vi "Reshape volume imaging data.vi"(0 "tdms file ref":refnum<k34>, 1 "TDMS file path & name":path=path "C:/Users/Theo/Desktop/Datasets/140401_17_44_08-rig 3 debugging/Functional imaging TDMS data files/001.tdms", 5 "All header parameters":T1={"Imaging Protocol"=enum."AOL Z-Stack", "Number of POI"=0, "Number of Miniscans"=0, "Number of Trials"=0, "Number of Cycles "=0, "# Averaged Frames"=0, "Laser power (%)"=0, "Pockels"=0.0, "Acquisition Length (sec)"=0.0, "Fill time (us)"=0.0, "POI Dwell time (us)"=0.0, "Miniscan Dwell time per pixel (us)"=0.0, "PMT 1"=0.0, "PMT 2"=0.0, "Back Apperture"=0.0, "Zoom"=0.0, "Frame Size"=200, "Center Frequency"=0.0, "Field of View"=0.0, "DwellTime (us)"=0.0, "Wavelength (nm)"=0.0, "AOL Z"=0.0, "AOL Mode"=enum."Raster", "GridXY"=0.0, "GridZ"=0.0, "TriggerDelay (sec)"=0.0, "Number of Pixels in Miniscan"=0, "Experiment folder path"=path "", "X centre"=0.0, "Y centre"=0.0, "Angle (degrees)"=0.0, "Plane Mode"=0, "Software version"=0.0, "Objective"="Olympus  20X", "MotorZ Calibration"=0, "Pockels Calibration"=0, "Threshold"=[], "Video length (sec)"=0.0, "Frame rate (fps)"=0, "Rectangle ROI length (pixels)"=0, "Rectangle ROI height (pixels)"=0} {"Pockels" format="%#.6g"; "Software version" format="%#.6g"; "Plane Mode" items=["XY Plane"]; "Angle (degrees)" format="%#.6g"; "Frame Size" items=["100X100"=100, "128X128"=128, "200X200"=200, "256X256"=256, "512X512"=512, "1024x1024"=1024, "2048x2048"=2048]; "Back Apperture" format="%#.6g"; "PMT 2" format="%#.6g"; "PMT 1" format="%#.6g"; "Miniscan Dwell time per pixel (us)" format="%#.6g"; "Zoom" format="%#.6g"; "POI Dwell time (us)" format="%#.6g"; "Acquisition Length (sec)" format="%#.6g"; "Fill time (us)" format="%#.6g"}, 11 "error in (no error)":errorcluster, 12 "Channel to process":enum16{"Red", "Green", "Both"}(ring)) -> (4 "tdms file out":refnum<k34>, 6 "Single channel data":u16[](array[numeric]), 8 "Channel 4D data":u16[][][][](array[numeric]), 10 "Volumetric parameters":T7, 14 "Angles (deg)":dbl[](array[numeric]), 15 "error out":errorcluster)   [LabVIEW 2013]
uses:
  User Interface/Visualisation/Functional Imaging Viewer/SubVIs/Experiment header interface/Typedefs/Header parameters cluster-ALL.ctl
  Typedefs/Imaging Protocols enum.ctl
  Typedefs/Frame Size.ctl
  Typedefs/AOL modes.ctl
  Typedefs/Plane Mode.ctl
  Typedefs/Objective selector control enum.ctl
panel:
  out "Points in each volume or trial (fractional)":dbl
  out "Points Mismatch":bool
  out "Resulting number of points":i32
  out "Points in each volume or trial":i32
  out "Points in all volumes":i32
  out "Channel size(s)":i32[](array[numeric])
  # "<---This should be an integer. If it is not review the logic inside this VI is suitable"
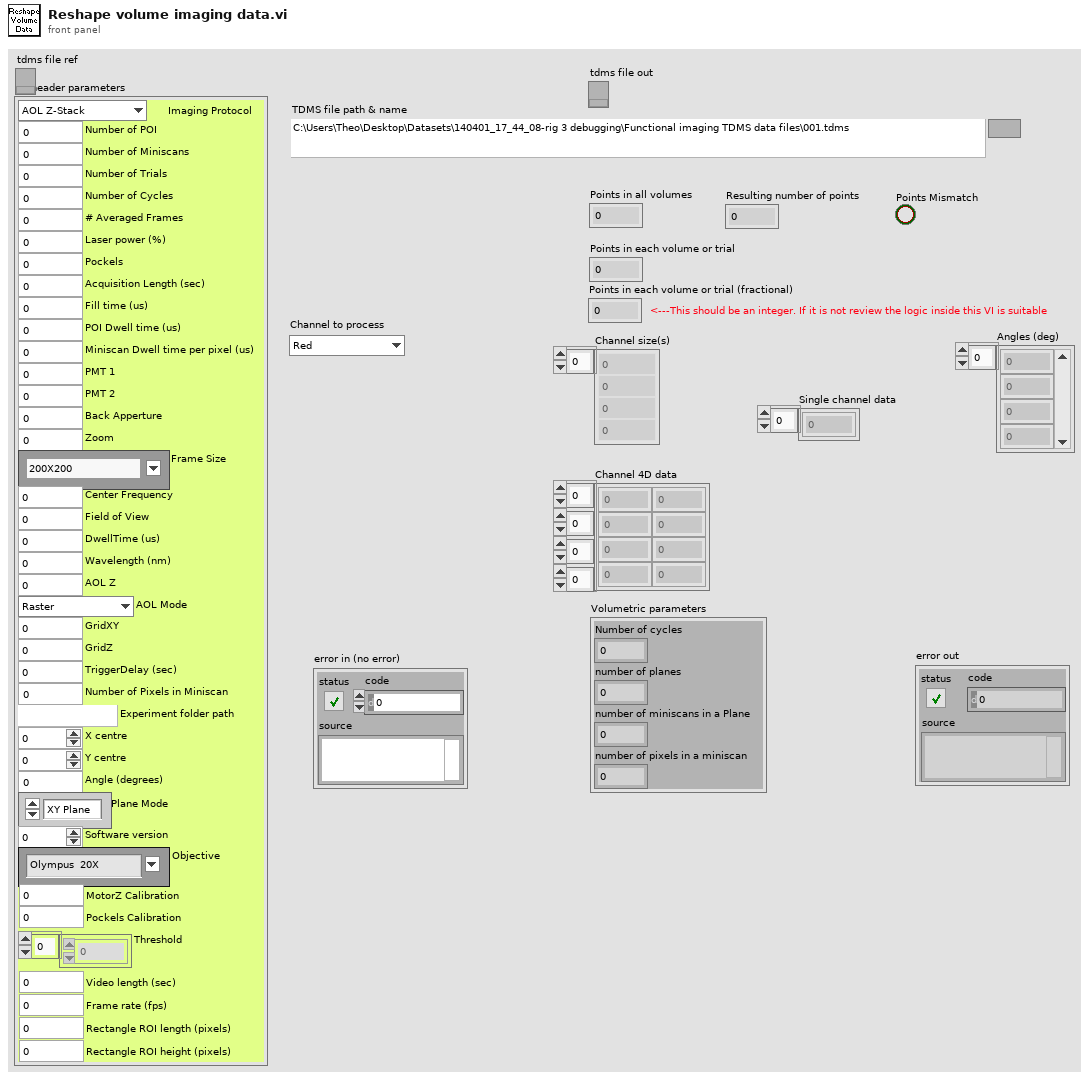
[diagram p1: front panel]
types:
  T1 = typedef "Header parameters cluster-ALL.ctl" = cluster{"Imaging Protocol":T2, "Number of POI":u16, "Number of Miniscans":u16, "Number of Trials":u16, "Number of Cycles ":u64, "# Averaged Frames":u16, "Laser power (%)":u8, "Pockels":dbl, "Acquisition Length (sec)":dbl, "Fill time (us)":dbl, "POI Dwell time (us)":dbl, "Miniscan Dwell time per pixel (us)":dbl, "PMT 1":dbl, "PMT 2":dbl, "Back Apperture":dbl, "Zoom":dbl, "Frame Size":T3, "Center Frequency":dbl, "Field of View":dbl, "DwellTime (us)":dbl, "Wavelength (nm)":dbl, "AOL Z":dbl, "AOL Mode":T4, "GridXY":dbl, "GridZ":dbl, "TriggerDelay (sec)":dbl, "Number of Pixels in Miniscan":u16, "Experiment folder path":path, "X centre":dbl, "Y centre":dbl, "Angle (degrees)":dbl, "Plane Mode":T5, "Software version":dbl, "Objective":T6, "MotorZ Calibration":u32, "Pockels Calibration":u32, "Threshold":u16[], "Video length (sec)":dbl, "Frame rate (fps)":u8, "Rectangle ROI length (pixels)":u16, "Rectangle ROI height (pixels)":u16}
  T2 = typedef "Imaging Protocols enum.ctl" = enum16{"AOL Z-Stack", "Motor Z Stack", "Functional Acquisition", "Single Plane Acquisition", "Volume Acquisition", "Live Imaging", "Live Plane Imaging", "Live Volume Imaging"}
  T3 = typedef "Frame Size.ctl" = u16
  T4 = typedef "AOL modes.ctl" = enum16{"Raster", "Structural", "Pointing", "Mini Scan", "Alignment"}
  T5 = typedef "Plane Mode.ctl" = u16
  T6 = typedef "Objective selector control enum.ctl" = string
  T7 = cluster{"Number of cycles":i32, "number of planes":i32, "number of miniscans in a Plane":i32, "number of pixels in a miniscan":i32}
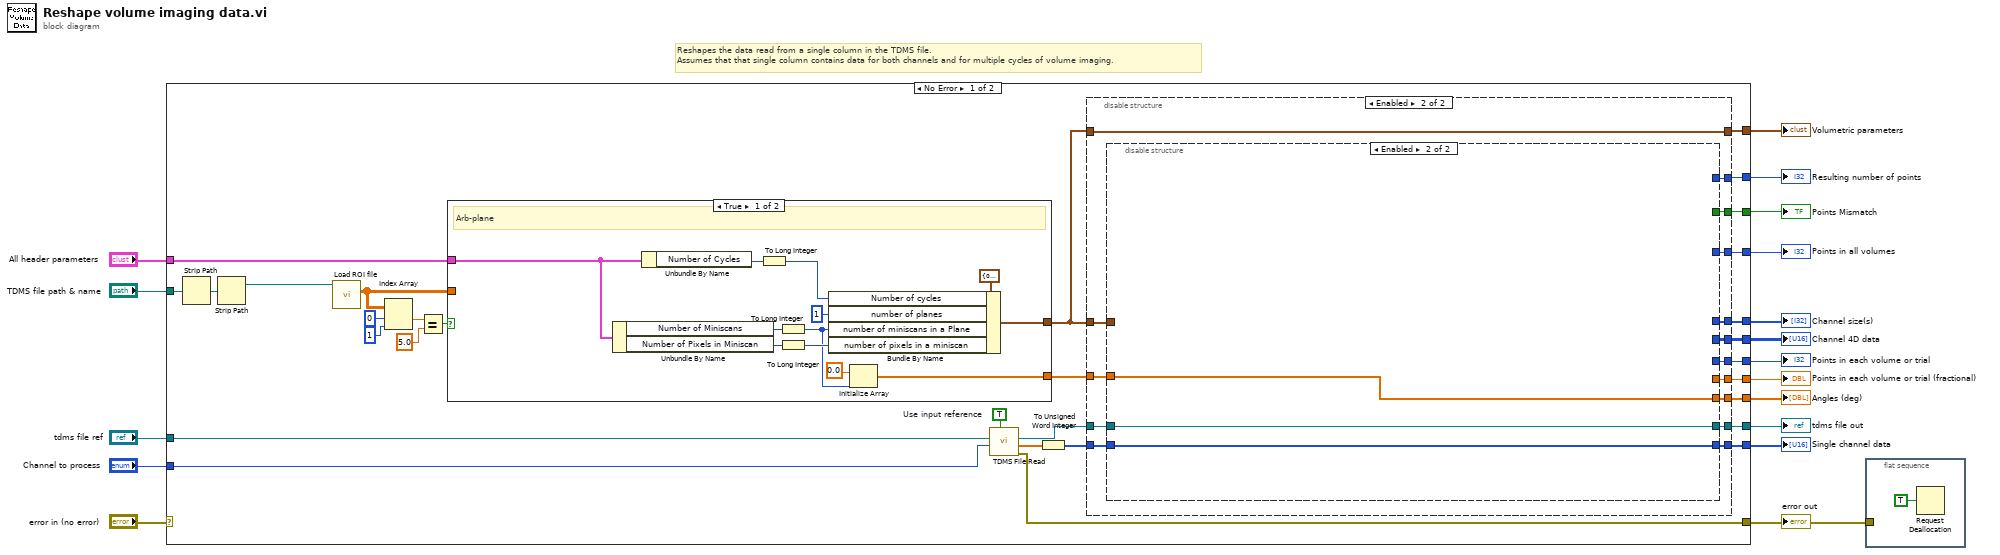
[diagram p0: block diagram]
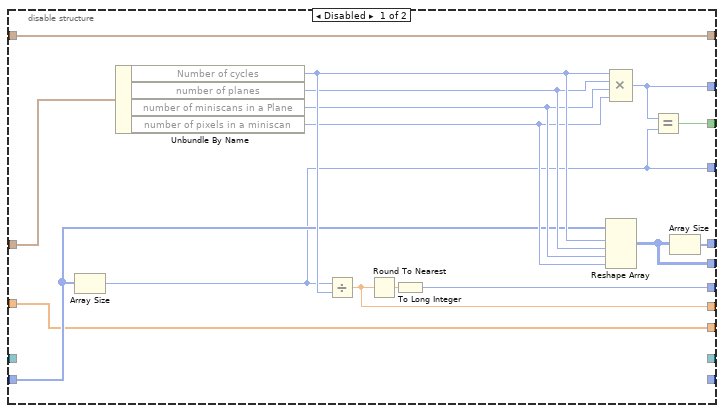
[diagram p2: hidden frame]
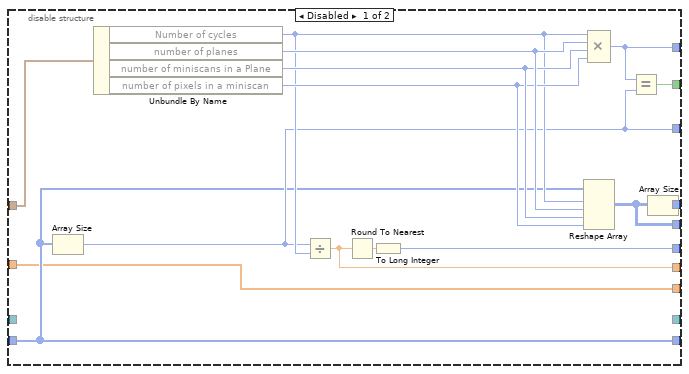
[diagram p3: hidden frame]
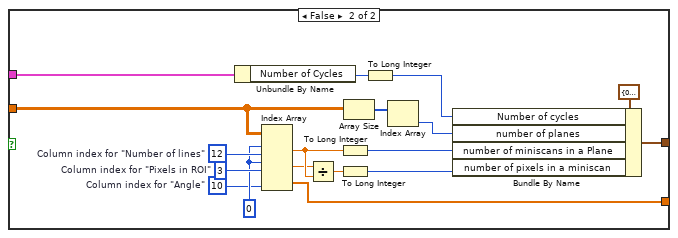
[diagram p4: hidden frame]
diagram:
  # "Reshapes the data read from a single column in the TDMS file.\nAssumes that that single column contains data for both channels and for multiple cycles of volume imaging."
  n1 = case shown="No Error" "error in (no error)" {
    selector: "error in (no error)" -> [_ w127]
    tunnel: [w47 _] -> w17
    tunnel: "TDMS file path & name" -> [w41 _]
    tunnel: [w46 _] -> w15
    tunnel: [w45 _] -> w14
    tunnel: [w44 _] -> w13
    tunnel: [w40 w127] -> w11
    tunnel: "All header parameters" -> [w33 _]
    tunnel: [w23 _] -> w9
    tunnel: [w27 _] -> w10
    tunnel: [w31 _] -> w7
    tunnel: [w30 _] -> w6
    tunnel: [w29 _] -> w5
    tunnel: "Channel to process" -> [w26 _]
    tunnel: [w25 _] -> w3
    tunnel: "tdms file ref" -> [w21 _]
    tunnel: [w18 _] -> w1
    frame No Error {
      w22 = TRUE  # Use input reference
      n2 = Strip Path(path=w41) -> (stripped path=w42:path)  [unwired: 1 out]
      n3 = Strip Path(path=w42) -> (stripped path=w43:path)  [unwired: 1 out]
      n4 = call "Load ROI file.vi"("Experiment data folder path"=w43) -> ("ROI Data (header removed)"=w39:dbl[][])  [unwired: 7 in, 3 out]
      n5 = Index Array(array=w39, index (row)=0, index (col)=1 ("disabled index (col)")) -> (element=w36:dbl)
      n6 = Equal?(x=w36, y=5.0) -> (x = y?=w34:bool)
      n7 = case shown="True" w34 {
        tunnel: [w108 w122] -> w24
        tunnel: [w104 w113] -> w28
        tunnel: w39 -> [_ w114]
        tunnel: w33 -> [w100 w110]
        frame True {
          # "Arb-plane"
          n8 = Unbundle By Name(w100) -> ("Number of Miniscans"=w99:u16, "Number of Pixels in Miniscan"=w98:u16)
          n9 = Unbundle By Name(w100) -> ("Number of Cycles"=w102:u64)
          n10 = To Long Integer(number=w102) -> (32bit integer=w101:i32)
          n11 = To Long Integer(number=w99) -> (32bit integer=w103:i32)
          n12 = To Long Integer(number=w98) -> (32bit integer=w106:i32)
          n13 = Bundle By Name(cluster=T7 {"Number of cycles"=0, "number of planes"=0, "number of miniscans in a Plane"=0, "number of pixels in a miniscan"=0} ("Parameters Cluster"), "Number of cycles"=w101, "number of planes"=1, "number of miniscans in a Plane"=w103, "number of pixels in a miniscan"=w106) -> (w108:T7)
          n14 = Initialize Array(0.0 ("element"), w103) -> (w104:dbl[])
        }
        frame False {
          w119 = 10  # Column index for "Angle"
          w120 = 0 ("disabled index (row)")
          w125 = 3  # Column index for "Pixels in ROI"
          w126 = 12  # Column index for "Number of lines"
          n15 = Unbundle By Name(w110) -> ("Number of Cycles"=w112:u64)
          n16 = Index Array(array=w114, index (row) #1=w120, index (col) #1=w126, index (row) #2=w120, index (col) #2=w125, index (col) #3=w119) -> (element #1=w118:dbl, element #2=w117:dbl, element #3=w113:dbl[])  [unwired: 1 in]
          n17 = Divide(x=w117, y=w118) -> (x/y=w121:dbl)
          n18 = To Long Integer(number=w118) -> (32bit integer=w116:i32)
          n19 = To Long Integer(number=w121) -> (32bit integer=w115:i32)
          n20 = Array Size(array=w114) -> (size(s)=w124:i32[])
          n21 = To Long Integer(number=w112) -> (32bit integer=w111:i32)
          n22 = Index Array(array=w124) -> (element=w123:i32)  [unwired: 1 in]
          n23 = Bundle By Name(cluster=T7 {"Number of cycles"=0, "number of planes"=0, "number of miniscans in a Plane"=0, "number of pixels in a miniscan"=0} ("Parameters Cluster"), "Number of cycles"=w111, "number of planes"=w123, "number of miniscans in a Plane"=w116, "number of pixels in a miniscan"=w115) -> (w122:T7)
        }
      }
      n24 = call "TDMS File Read.vi"("Use input reference (F)"=w22, "Channel to load"=w26, "tdms file ref"=w21) -> ("Error Out"=w40:errorcluster, "Single channel data"=w20:dbl[], "tdms file out"=w19:refnum<k34>)  [unwired: 5 in, 1 out]
      n25 = To Unsigned Word Integer(number=w20) -> (unsigned 16bit integer=w32:u16[])
      n26 = disable-structure shown="Enabled" {
        disable-tunnel: [w63 w78] -> w47
        disable-tunnel: [w61 w77] -> w46
        disable-tunnel: [w60 w76] -> w45
        disable-tunnel: [w59 w75] -> w44
        disable-tunnel: w24 -> [w48 w71]
        disable-tunnel: w32 -> [w54 w70]
        disable-tunnel: [w53 w74] -> w31
        disable-tunnel: [w52 w73] -> w30
        disable-tunnel: [w51 w72] -> w29
        disable-tunnel: w28 -> [w50 w68]
        disable-tunnel: [w50 w67] -> w27
        disable-tunnel: [_ w69] -> w25
        disable-tunnel: w24 -> [w49 w66]
        disable-tunnel: [w49 w66] -> w23
        disable-tunnel: w19 -> [_ w65]
        disable-tunnel: [_ w64] -> w18
        frame Disabled {
          n27 = Array Size(array=w54) -> (size(s)=w51:i32)
          n28 = Unbundle By Name(w48) -> ("Number of cycles"=w58:i32, "number of planes"=w57:i32, "number of miniscans in a Plane"=w56:i32, "number of pixels in a miniscan"=w55:i32)
          n29 = Divide(x=w51, y=w58) -> (x/y=w52:dbl)
          n30 = Round To Nearest(number=w52) -> (nearest integer value=w62:dbl)
          n31 = To Long Integer(number=w62) -> (32bit integer=w53:i32)
          n32 = Reshape Array(w54, w58, w57, w56, w55) -> (w59:u16[][][][])
          n33 = Compound Arithmetic op=MULTIPLY(w58, w57, w56, w55) -> (w61:i32)
          n34 = Equal?(x=w61, y=w51) -> (x = y?=w60:bool)
          n35 = Array Size(array=w59) -> (size(s)=w63:i32[])
        }
        frame Enabled {
          n36 = disable-structure shown="Enabled" {
            disable-tunnel: [w93 _] -> w78
            disable-tunnel: [w91 _] -> w77
            disable-tunnel: [w90 _] -> w76
            disable-tunnel: [w89 _] -> w75
            disable-tunnel: [w85 _] -> w74
            disable-tunnel: [w84 _] -> w73
            disable-tunnel: [w82 _] -> w72
            disable-tunnel: w71 -> [w81 _]
            disable-tunnel: w70 -> [w80 w96]
            disable-tunnel: [w80 w96] -> w69
            disable-tunnel: w68 -> [w79 w95]
            disable-tunnel: [w79 w95] -> w67
            disable-tunnel: w65 -> [_ w94]
            disable-tunnel: [_ w94] -> w64
            frame Disabled {
              n37 = Array Size(array=w80) -> (size(s)=w82:i32)
              n38 = Unbundle By Name(w81) -> ("Number of cycles"=w83:i32, "number of planes"=w88:i32, "number of miniscans in a Plane"=w87:i32, "number of pixels in a miniscan"=w86:i32)
              n39 = Divide(x=w82, y=w83) -> (x/y=w84:dbl)
              n40 = Round To Nearest(number=w84) -> (nearest integer value=w92:dbl)
              n41 = To Long Integer(number=w92) -> (32bit integer=w85:i32)
              n42 = Reshape Array(w80, w83, w88, w87, w86) -> (w89:u16[][][][])
              n43 = Compound Arithmetic op=MULTIPLY(w83, w88, w87, w86) -> (w91:i32)
              n44 = Equal?(x=w91, y=w82) -> (x = y?=w90:bool)
              n45 = Array Size(array=w89) -> (size(s)=w93:i32[])
            }
            frame Enabled {
            }
          }
        }
      }
    }
    frame Error {
    }
  }
  "Channel size(s)" <- w17
  "Resulting number of points" <- w15
  "Points Mismatch" <- w14
  "Channel 4D data" <- w13
  "error out" <- w11
  "Volumetric parameters" <- w9
  "Angles (deg)" <- w10
  "Points in each volume or trial" <- w7
  "Points in each volume or trial (fractional)" <- w6
  "Points in all volumes" <- w5
  "Single channel data" <- w3
  "tdms file out" <- w1
  n46 = flat-sequence {
    tunnel: w11 -> [_]
    frame #0 {
      n47 = Request Deallocation(TRUE ("flag")) -> ()
    }
  }
